vi "Dresden Edit Recipe(in).vi"() -> ()   [LabVIEW 2009] (continued)
              n372 = local write "R_Recipe_type_selection"(enum32{"Single Recipe", "Combination Sputter"}."Combination Sputter" ("R_Recipe_type_selection")) -> ()
              n373 = property on="R Web speed(cm/min)" class="DigNum (strict)"("DisabledEnum"=T5."Disabled and Grayed Out" ("Disabled")) -> ()  [unwired: 2 in, 2 out]
            }
          }
          n374 = Mantissa & Exponent(0:w608) -> (2:w601:dbl)  [unwired: 1 out]
          n375 = Equal?(x="Active", y=w267) -> (x = y?=w269:bool)
          n376 = local write "R_Target Thickness Value"(w495) -> ()
          n377 = local write "R_Duration"(w494) -> ()
          n378 = local write "R Maximum diameter"(w500) -> ()
          n379 = local write "R Minimum diameter"(w501) -> ()
          n380 = local write "R Web thickness"(w499) -> ()
          n381 = local write "R Web speed(cm/min)"(w498) -> ()
          n382 = local write "R Tension Value"(w497) -> ()
          n383 = local write "R  Total length"(w496) -> ()
          n384 = case shown="True" w269 {
            frame #0 {
              n385 = local write "R Single DC Step2 Coating Power Active"(FALSE ("R Single DC Step1 Coating Power Active")) -> ()
            }
            frame #1 {
              n386 = local write "R Single DC Step2 Coating Power Active"(TRUE ("R Single DC Step1 Coating Power Active")) -> ()
            }
          }
          n387 = case shown="True" w271 {
            frame #0 {
              n388 = local write "R Single DC Step1 Coating Power Active"(FALSE ("R Single DC Step1 Coating Power Active")) -> ()
            }
            frame #1 {
              n389 = local write "R Single DC Step1 Coating Power Active"(TRUE ("R Single DC Step1 Coating Power Active")) -> ()
            }
          }
          n390 = case shown="1" w601 {
            frame #0 {
            }
            frame #1 {
              n391 = local write "R_DC_Chamber_selection"(enum32{"Chamber II", "Chamber III"}."Chamber II" ("R_DC_Chamber_selection")) -> ()
            }
            frame #2 {
              n392 = local write "R_DC_Chamber_selection"(enum32{"Chamber II", "Chamber III"}."Chamber III" ("R_DC_Chamber_selection")) -> ()
            }
          }
          n393 = stacked-sequence {
            frame #0 {
            }
          }
          n394 = stacked-sequence {
            frame #0 {
            }
          }
          n395 = stacked-sequence {
            frame #0 {
            }
          }
          n396 = stacked-sequence {
            frame #0 {
              # "Recipe Parameters"
            }
          }
        }
        frame #1 {
        }
      }
    }
    frame #4 {
      n397 = local read "Recipe_cancel"() -> (w818:bool)
      n398 = case shown="False" w818 {
        frame #0 {
          n399 = Wait (ms)(milliseconds to wait=u32 1000) -> ()  [unwired: 1 out]
        }
        frame #1 {
        }
      }
    }
    frame #5 {
      n400 = local read "Recipe_cancel"() -> (w821:bool)
      n401 = case shown="False" w821 {
        tunnel: [w822 FALSE] -> w820
        frame #0 {
          n402 = while {
            tunnel: [w851] -> w822
            stop <- w851 stop-if-true
            n403 = local read "R Single DC Step1 Coating Power Active"() -> (w850:bool)
            n404 = local read "R Single RF Step4 Coating Power Active"() -> (w838:bool)
            n405 = local read "R Single DC Step4 Coating Power Active"() -> (w847:bool)
            n406 = local read "R Single DC Step2 Coating Power Active"() -> (w849:bool)
            n407 = local read "R Single RF Step3 Coating Power Active"() -> (w839:bool)
            n408 = local read "R Single RF Step1 Coating Power Active"() -> (w841:bool)
            n409 = local read "R Single DC Step3 Coating Power Active"() -> (w848:bool)
            n410 = local read "R Single RF Step5 Coating Power Active"() -> (w837:bool)
            n411 = local read "R Single RF Step9 Coating Power Active"() -> (w836:bool)
            n412 = local read "R_Recipe_type_selection"() -> (w823:enum32{"Single Recipe", "Combination Sputter"})
            n413 = local read "R Single RF Step2 Coating Power Active"() -> (w840:bool)
            n414 = case shown="\"Combination Sputter\"" w823 {
              frame #0 {
                n415 = local read "Web_selection_tab"() -> (w1019:T4)
                n416 = Equal?(x=w1019, y=0) -> (x = y?=w1018:bool)
                n417 = case shown="True" w1018 {
                  frame #0 {
                  }
                  frame #1 {
                    w1021 = T5."Enabled" ("Disabled")
                    n418 = property on="R Minimum diameter" class="DigNum (strict)"("DisabledEnum"=w1021) -> ()  [unwired: 2 in, 2 out]
                    n419 = property on="R Maximum diameter" class="DigNum (strict)"("DisabledEnum"=w1021) -> ()  [unwired: 2 in, 2 out]
                    n420 = property on="R Web thickness" class="DigNum (strict)"("DisabledEnum"=w1021) -> ()  [unwired: 2 in, 2 out]
                    n421 = property on="R Web speed(cm/min)" class="DigNum (strict)"("DisabledEnum"=w1021) -> ()  [unwired: 2 in, 2 out]
                    n422 = property on="R Tension Value" class="DigNum (strict)"("DisabledEnum"=w1021) -> ()  [unwired: 2 in, 2 out]
                    n423 = property on="R_Single Microwave Time" class="DigNum (strict)"("DisabledEnum"=T5."Disabled and Grayed Out" ("Disabled")) -> ()  [unwired: 2 in, 2 out]
                  }
                }
              }
              frame #1 {
                n424 = local read "R_Web_selection"() -> (w1024:enum32{"Web", "Other"})
                n425 = Equal?(x=w1024, y=0) -> (x = y?=w1025:bool)
                n426 = case shown="True" w1025 {
                  frame #0 {
                  }
                  frame #1 {
                    w1027 = T5."Enabled" ("Disabled")
                    n427 = local write "R Web speed(cm/min)"(0.0 ("R Web speed(cm/min)")) -> ()
                    n428 = property on="R Tension Value" class="DigNum (strict)"("DisabledEnum"=w1027) -> ()  [unwired: 2 in, 2 out]
                    n429 = property on="R Minimum diameter" class="DigNum (strict)"("DisabledEnum"=w1027) -> ()  [unwired: 2 in, 2 out]
                    n430 = property on="R Maximum diameter" class="DigNum (strict)"("DisabledEnum"=w1027) -> ()  [unwired: 2 in, 2 out]
                    n431 = property on="R Web thickness" class="DigNum (strict)"("DisabledEnum"=w1027) -> ()  [unwired: 2 in, 2 out]
                    n432 = property on="R Web speed(cm/min)" class="DigNum (strict)"("DisabledEnum"=T5."Disabled and Grayed Out" ("Disabled")) -> ()  [unwired: 2 in, 2 out]
                  }
                }
              }
            }
            n433 = case shown="True" w850 {
              frame #0 {
              }
              frame #1 {
                n434 = local read "R Single DC Step2 Coating Power Active"() -> (w1157:bool)
                n435 = case shown="False" w1157 {
                  frame #0 {
                    w1158 = 0.0 ("Target Clean Power")
                    w1159 = T5."Disabled and Grayed Out" ("Disabled")
                    n436 = local write "R Single DC Step2 Coating Power"(w1158) -> ()
                    n437 = local write "R Single DC Interval length2"(w1158) -> ()
                    n438 = property on="R Single DC Interval length2" class="DigNum (strict)"("DisabledEnum"=w1159) -> ()  [unwired: 2 in, 2 out]
                    n439 = property on="R Single DC Step2 Coating Power" class="DigNum (strict)"("DisabledEnum"=w1159) -> ()  [unwired: 2 in, 2 out]
                  }
                  frame #1 {
                    w1160 = T5."Enabled" ("Disabled")
                    n440 = property on="R Single DC Step2 Coating Power" class="DigNum (strict)"("DisabledEnum"=w1160) -> ()  [unwired: 2 in, 2 out]
                    n441 = property on="R Single DC Interval length2" class="DigNum (strict)"("DisabledEnum"=w1160) -> ()  [unwired: 2 in, 2 out]
                  }
                }
              }
            }
            n442 = local read "R_Recipe_type_selection"() -> (w989:enum32{"Single Recipe", "Combination Sputter"})
            n443 = case shown="False" w838 {
              frame #0 {
                w1098 = FALSE ("R Single RF Step3 Coating Power Active")
                n444 = local write "R Single RF Step5 Coating Power Active"(w1098) -> ()
                n445 = local write "R Single RF Step6 Coating Power Active"(w1098) -> ()
                n446 = local write "R Single RF Step7 Coating Power Active"(w1098) -> ()
                n447 = local write "R Single RF Step8 Coating Power Active"(w1098) -> ()
                n448 = local write "R Single RF Step9 Coating Power Active"(w1098) -> ()
                n449 = local write "R Single RF Step10 Coating Power Active"(w1098) -> ()
              }
              frame #1 {
                n450 = local read "R Single RF Step5 Coating Power Active"() -> (w1099:bool)
                n451 = case shown="False" w1099 {
                  frame #0 {
                    w1101 = T5."Disabled and Grayed Out" ("Disabled")
                    w1100 = 0.0 ("Target Clean Power")
                    n452 = local write "R Single RF Step5 Coating Power"(w1100) -> ()
                    n453 = local write "R Single RF Interval length5"(w1100) -> ()
                    n454 = property on="R Single RF Interval length5" class="DigNum (strict)"("DisabledEnum"=w1101) -> ()  [unwired: 2 in, 2 out]
                    n455 = property on="R Single RF Step5 Coating Power" class="DigNum (strict)"("DisabledEnum"=w1101) -> ()  [unwired: 2 in, 2 out]
                  }
                  frame #1 {
                    w1102 = T5."Enabled" ("Disabled")
                    n456 = property on="R Single RF Step5 Coating Power" class="DigNum (strict)"("DisabledEnum"=w1102) -> ()  [unwired: 2 in, 2 out]
                    n457 = property on="R Single RF Interval length5" class="DigNum (strict)"("DisabledEnum"=w1102) -> ()  [unwired: 2 in, 2 out]
                  }
                }
              }
            }
            n458 = local read "R_Recipe_type_selection"() -> (w858:enum32{"Single Recipe", "Combination Sputter"})
            n459 = case shown="False" w839 {
              frame #0 {
                w1103 = FALSE ("R Single RF Step3 Coating Power Active")
                n460 = local write "R Single RF Step4 Coating Power Active"(w1103) -> ()
                n461 = local write "R Single RF Step5 Coating Power Active"(w1103) -> ()
                n462 = local write "R Single RF Step6 Coating Power Active"(w1103) -> ()
                n463 = local write "R Single RF Step7 Coating Power Active"(w1103) -> ()
                n464 = local write "R Single RF Step8 Coating Power Active"(w1103) -> ()
                n465 = local write "R Single RF Step9 Coating Power Active"(w1103) -> ()
                n466 = local write "R Single RF Step10 Coating Power Active"(w1103) -> ()
              }
              frame #1 {
                n467 = local read "R Single RF Step4 Coating Power Active"() -> (w1104:bool)
                n468 = case shown="False" w1104 {
                  frame #0 {
                    w1106 = T5."Disabled and Grayed Out" ("Disabled")
                    w1105 = 0.0 ("Target Clean Power")
                    n469 = local write "R Single RF Interval length4"(w1105) -> ()
                    n470 = local write "R Single RF Step4 Coating Power"(w1105) -> ()
                    n471 = property on="R Single RF Step4 Coating Power" class="DigNum (strict)"("DisabledEnum"=w1106) -> ()  [unwired: 2 in, 2 out]
                    n472 = property on="R Single RF Interval length4" class="DigNum (strict)"("DisabledEnum"=w1106) -> ()  [unwired: 2 in, 2 out]
                  }
                  frame #1 {
                    w1107 = T5."Enabled" ("Disabled")
                    n473 = property on="R Single RF Step4 Coating Power" class="DigNum (strict)"("DisabledEnum"=w1107) -> ()  [unwired: 2 in, 2 out]
                    n474 = property on="R Single RF Interval length4" class="DigNum (strict)"("DisabledEnum"=w1107) -> ()  [unwired: 2 in, 2 out]
                  }
                }
              }
            }
            n475 = case shown="False" w849 {
              frame #0 {
                w1152 = FALSE ("R Single DC Step8 Coating Power Active")
                n476 = local write "R Single DC Step7 Coating Power Active"(w1152) -> ()
                n477 = local write "R Single DC Step8 Coating Power Active"(w1152) -> ()
                n478 = local write "R Single DC Step9 Coating Power Active"(w1152) -> ()
                n479 = local write "R Single DC Step10 Coating Power Active"(w1152) -> ()
                n480 = local write "R Single DC Step6 Coating Power Active"(w1152) -> ()
                n481 = local write "R Single DC Step3 Coating Power Active"(w1152) -> ()
                n482 = local write "R Single DC Step4 Coating Power Active"(w1152) -> ()
                n483 = local write "R Single DC Step5 Coating Power Active"(w1152) -> ()
              }
              frame #1 {
                n484 = local read "R Single DC Step3 Coating Power Active"() -> (w1153:bool)
                n485 = case shown="False" w1153 {
                  frame #0 {
                    w1154 = 0.0 ("Target Clean Power")
                    w1155 = T5."Disabled and Grayed Out" ("Disabled")
                    n486 = local write "R Single DC Step3 Coating Power"(w1154) -> ()
                    n487 = local write "R Single DC Interval length3"(w1154) -> ()
                    n488 = property on="R Single DC Interval length3" class="DigNum (strict)"("DisabledEnum"=w1155) -> ()  [unwired: 2 in, 2 out]
                    n489 = property on="R Single DC Step3 Coating Power" class="DigNum (strict)"("DisabledEnum"=w1155) -> ()  [unwired: 2 in, 2 out]
                  }
                  frame #1 {
                    w1156 = T5."Enabled" ("Disabled")
                    n490 = property on="R Single DC Step3 Coating Power" class="DigNum (strict)"("DisabledEnum"=w1156) -> ()  [unwired: 2 in, 2 out]
                    n491 = property on="R Single DC Interval length3" class="DigNum (strict)"("DisabledEnum"=w1156) -> ()  [unwired: 2 in, 2 out]
                  }
                }
              }
            }
            n492 = case shown="False" w847 {
              frame #0 {
                w1142 = FALSE ("R Single DC Step8 Coating Power Active")
                n493 = local write "R Single DC Step7 Coating Power Active"(w1142) -> ()
                n494 = local write "R Single DC Step8 Coating Power Active"(w1142) -> ()
                n495 = local write "R Single DC Step9 Coating Power Active"(w1142) -> ()
                n496 = local write "R Single DC Step10 Coating Power Active"(w1142) -> ()
                n497 = local write "R Single DC Step5 Coating Power Active"(w1142) -> ()
                n498 = local write "R Single DC Step6 Coating Power Active"(w1142) -> ()
              }
              frame #1 {
                n499 = local read "R Single DC Step5 Coating Power Active"() -> (w1143:bool)
                n500 = case shown="False" w1143 {
                  frame #0 {
                    w1144 = 0.0 ("Target Clean Power")
                    w1145 = T5."Disabled and Grayed Out" ("Disabled")
                    n501 = local write "R Single DC Step5 Coating Power"(w1144) -> ()
                    n502 = local write "R Single DC Interval length5"(w1144) -> ()
                    n503 = property on="R Single DC Step5 Coating Power" class="DigNum (strict)"("DisabledEnum"=w1145) -> ()  [unwired: 2 in, 2 out]
                    n504 = property on="R Single DC Interval length5" class="DigNum (strict)"("DisabledEnum"=w1145) -> ()  [unwired: 2 in, 2 out]
                  }
                  frame #1 {
                    w1146 = T5."Enabled" ("Disabled")
                    n505 = property on="R Single DC Step5 Coating Power" class="DigNum (strict)"("DisabledEnum"=w1146) -> ()  [unwired: 2 in, 2 out]
                    n506 = property on="R Single DC Interval length5" class="DigNum (strict)"("DisabledEnum"=w1146) -> ()  [unwired: 2 in, 2 out]
                  }
                }
              }
            }
            n507 = case shown="False" w848 {
              frame #0 {
                w1147 = FALSE ("R Single DC Step8 Coating Power Active")
                n508 = local write "R Single DC Step7 Coating Power Active"(w1147) -> ()
                n509 = local write "R Single DC Step8 Coating Power Active"(w1147) -> ()
                n510 = local write "R Single DC Step9 Coating Power Active"(w1147) -> ()
                n511 = local write "R Single DC Step10 Coating Power Active"(w1147) -> ()
                n512 = local write "R Single DC Step6 Coating Power Active"(w1147) -> ()
                n513 = local write "R Single DC Step5 Coating Power Active"(w1147) -> ()
                n514 = local write "R Single DC Step4 Coating Power Active"(w1147) -> ()
              }
              frame #1 {
                n515 = local read "R Single DC Step4 Coating Power Active"() -> (w1148:bool)
                n516 = case shown="False" w1148 {
                  frame #0 {
                    w1149 = 0.0 ("Target Clean Power")
                    w1150 = T5."Disabled and Grayed Out" ("Disabled")
                    n517 = local write "R Single DC Step4 Coating Power"(w1149) -> ()
                    n518 = local write "R Single DC Interval length4"(w1149) -> ()
                    n519 = property on="R Single DC Step4 Coating Power" class="DigNum (strict)"("DisabledEnum"=w1150) -> ()  [unwired: 2 in, 2 out]
                    n520 = property on="R Single DC Interval length4" class="DigNum (strict)"("DisabledEnum"=w1150) -> ()  [unwired: 2 in, 2 out]
                  }
                  frame #1 {
                    w1151 = T5."Enabled" ("Disabled")
                    n521 = property on="R Single DC Step4 Coating Power" class="DigNum (strict)"("DisabledEnum"=w1151) -> ()  [unwired: 2 in, 2 out]
                    n522 = property on="R Single DC Interval length4" class="DigNum (strict)"("DisabledEnum"=w1151) -> ()  [unwired: 2 in, 2 out]
                  }
                }
              }
            }
            n523 = case shown="True" w841 {
              frame #0 {
              }
              frame #1 {
                n524 = local read "R Single RF Step2 Coating Power Active"() -> (w1113:bool)
                n525 = case shown="False" w1113 {
                  frame #0 {
                    w1115 = T5."Disabled and Grayed Out" ("Disabled")
                    w1114 = 0.0 ("Target Clean Power")
                    n526 = local write "R Single RF Step2 Coating Power"(w1114) -> ()
                    n527 = local write "R Single RF Interval length2"(w1114) -> ()
                    n528 = property on="R Single RF Step2 Coating Power" class="DigNum (strict)"("DisabledEnum"=w1115) -> ()  [unwired: 2 in, 2 out]
                    n529 = property on="R Single RF Interval length2" class="DigNum (strict)"("DisabledEnum"=w1115) -> ()  [unwired: 2 in, 2 out]
                  }
                  frame #1 {
                    w1116 = T5."Enabled" ("Disabled")
                    n530 = property on="R Single RF Step2 Coating Power" class="DigNum (strict)"("DisabledEnum"=w1116) -> ()  [unwired: 2 in, 2 out]
                    n531 = property on="R Single RF Interval length2" class="DigNum (strict)"("DisabledEnum"=w1116) -> ()  [unwired: 2 in, 2 out]
                  }
                }
              }
            }
            n532 = local read "R Single RF Step1 Coating Power Active"() -> (w997:bool)
            n533 = case shown="False" w840 {
              frame #0 {
                w1108 = FALSE ("R Single RF Step3 Coating Power Active")
                n534 = local write "R Single RF Step3 Coating Power Active"(w1108) -> ()
                n535 = local write "R Single RF Step4 Coating Power Active"(w1108) -> ()
                n536 = local write "R Single RF Step5 Coating Power Active"(w1108) -> ()
                n537 = local write "R Single RF Step6 Coating Power Active"(w1108) -> ()
                n538 = local write "R Single RF Step7 Coating Power Active"(w1108) -> ()
                n539 = local write "R Single RF Step8 Coating Power Active"(w1108) -> ()
                n540 = local write "R Single RF Step9 Coating Power Active"(w1108) -> ()
                n541 = local write "R Single RF Step10 Coating Power Active"(w1108) -> ()
              }
              frame #1 {
                n542 = local read "R Single RF Step3 Coating Power Active"() -> (w1109:bool)
                n543 = case shown="False" w1109 {
                  frame #0 {
                    w1111 = T5."Disabled and Grayed Out" ("Disabled")
                    w1110 = 0.0 ("Target Clean Power")
                    n544 = local write "R Single RF Step3 Coating Power"(w1110) -> ()
                    n545 = local write "R Single RF Interval length3"(w1110) -> ()
                    n546 = property on="R Single RF Step3 Coating Power" class="DigNum (strict)"("DisabledEnum"=w1111) -> ()  [unwired: 2 in, 2 out]
                    n547 = property on="R Single RF Interval length3" class="DigNum (strict)"("DisabledEnum"=w1111) -> ()  [unwired: 2 in, 2 out]
                  }
                  frame #1 {
                    w1112 = T5."Enabled" ("Disabled")
                    n548 = property on="R Single RF Step3 Coating Power" class="DigNum (strict)"("DisabledEnum"=w1112) -> ()  [unwired: 2 in, 2 out]
                    n549 = property on="R Single RF Interval length3" class="DigNum (strict)"("DisabledEnum"=w1112) -> ()  [unwired: 2 in, 2 out]
                  }
                }
              }
            }
            n550 = case shown="False" w837 {
              frame #0 {
                w1093 = FALSE ("R Single RF Step3 Coating Power Active")
                n551 = local write "R Single RF Step6 Coating Power Active"(w1093) -> ()
                n552 = local write "R Single RF Step7 Coating Power Active"(w1093) -> ()
                n553 = local write "R Single RF Step8 Coating Power Active"(w1093) -> ()
                n554 = local write "R Single RF Step9 Coating Power Active"(w1093) -> ()
                n555 = local write "R Single RF Step10 Coating Power Active"(w1093) -> ()
              }
              frame #1 {
                n556 = local read "R Single RF Step6 Coating Power Active"() -> (w1094:bool)
                n557 = case shown="False" w1094 {
                  frame #0 {
                    w1095 = 0.0 ("Target Clean Power")
                    w1096 = T5."Disabled and Grayed Out" ("Disabled")
                    n558 = property on="R Single RF Interval length6" class="DigNum (strict)"("DisabledEnum"=w1096) -> ()  [unwired: 2 in, 2 out]
                    n559 = property on="R Single RF Step6 Coating Power" class="DigNum (strict)"("DisabledEnum"=w1096) -> ()  [unwired: 2 in, 2 out]
                    n560 = local write "R Single RF Step6 Coating Power"(w1095) -> ()
                    n561 = local write "R Single RF Interval length6"(w1095) -> ()
                  }
                  frame #1 {
                    w1097 = T5."Enabled" ("Disabled")
                    n562 = property on="R Single RF Step6 Coating Power" class="DigNum (strict)"("DisabledEnum"=w1097) -> ()  [unwired: 2 in, 2 out]
                    n563 = property on="R Single RF Interval length6" class="DigNum (strict)"("DisabledEnum"=w1097) -> ()  [unwired: 2 in, 2 out]
                  }
                }
              }
            }
            n564 = case shown="False" w836 {
              frame #0 {
                n565 = local write "R Single RF Step10 Coating Power Active"(FALSE ("R Single RF Step3 Coating Power Active")) -> ()
              }
              frame #1 {
                n566 = local read "R Single RF Step10 Coating Power Active"() -> (w1089:bool)
                n567 = case shown="False" w1089 {
                  frame #0 {
                    w1090 = 0.0 ("Target Clean Power")
                    w1091 = T5."Disabled and Grayed Out" ("Disabled")
                    n568 = local write "R Single RF Step10 Coating Power"(w1090) -> ()
                    n569 = local write "R Single RF Interval length10"(w1090) -> ()
                    n570 = property on="R Single RF Step10 Coating Power" class="DigNum (strict)"("DisabledEnum"=w1091) -> ()  [unwired: 2 in, 2 out]
                    n571 = property on="R Single RF Interval length10" class="DigNum (strict)"("DisabledEnum"=w1091) -> ()  [unwired: 2 in, 2 out]
                  }
                  frame #1 {
                    w1092 = T5."Enabled" ("Disabled")
                    n572 = property on="R Single RF Step10 Coating Power" class="DigNum (strict)"("DisabledEnum"=w1092) -> ()  [unwired: 2 in, 2 out]
                    n573 = property on="R Single RF Interval length10" class="DigNum (strict)"("DisabledEnum"=w1092) -> ()  [unwired: 2 in, 2 out]
                  }
                }
              }
            }
            n574 = local read "R_Simple_Coating Type Selection"() -> (w1005:T2)
            n575 = local read "R Single DC Step1 Coating Power Active"() -> (w998:bool)
            n576 = local read "R_Web_selection"() -> (w1010:enum32{"Web", "Other"})
            n577 = local read "R_Recipe_type_selection"() -> (w1006:enum32{"Single Recipe", "Combination Sputter"})
            n578 = Wait Until Next ms Multiple(millisecond multiple=u32 50) -> ()  [unwired: 1 out]
            n579 = local read "R Single DC Step1 Coating Power Active"() -> (w981:bool)
            n580 = local read "R Single DC Step4 Coating Power Active"() -> (w973:bool)
            n581 = local read "R Single DC Step3 Coating Power Active"() -> (w975:bool)
            n582 = local read "R Single DC Step2 Coating Power Active"() -> (w979:bool)
            n583 = local read "R Single DC Step5 Coating Power Active"() -> (w965:bool)
            n584 = local read "R Single DC Step6 Coating Power Active"() -> (w964:bool)
            n585 = local read "R Single DC Step7 Coating Power Active"() -> (w963:bool)
            n586 = local read "R Single DC Step10 Coating Power Active"() -> (w960:bool)
            n587 = local read "R Single RF Step7 Coating Power Active"() -> (w925:bool)
            n588 = local read "R Single DC Step8 Coating Power Active"() -> (w962:bool)
            n589 = local read "R Single DC Step9 Coating Power Active"() -> (w961:bool)
            n590 = local read "R Single RF Step9 Coating Power Active"() -> (w923:bool)
            n591 = local read "R Single RF Step10 Coating Power Active"() -> (w922:bool)
            n592 = local read "R Single RF Ramp up"() -> (w995:bool)
            n593 = local read "R Single RF Step1 Coating Power Active"() -> (w940:bool)
            n594 = local read "R Single RF Step2 Coating Power Active"() -> (w930:bool)
            n595 = local read "R Single RF Step3 Coating Power Active"() -> (w929:bool)
            n596 = local read "R Single RF Step4 Coating Power Active"() -> (w928:bool)
            n597 = local read "R Single RF Step5 Coating Power Active"() -> (w927:bool)
            n598 = local read "R Single RF Step6 Coating Power Active"() -> (w926:bool)
            n599 = local read "R Single RF Step8 Coating Power Active"() -> (w924:bool)
            n600 = local read "R Single RF Ramp down"() -> (w996:bool)
            n601 = Equal?(x=w989, y=0) -> (x = y?=w859:bool)
            n602 = Equal?(x=w858, y=1) -> (x = y?=w856:bool)
            n603 = case shown="True" "OK" {
              tunnel: [FALSE w1310] -> w853
              frame #0 {
              }
              frame #1 {
                # "TENSION IS NOT LOWER THAN 5\nTENSION IS NOT BIGGER THAN10"
                # "92"
                # "91"
                # "2"
                # "1"
                n604 = local read "R_Web_selection"() -> (w1306:enum32{"Web", "Other"})
                n605 = local read "R_Recipe_type_selection"() -> (w1328:enum32{"Single Recipe", "Combination Sputter"})
                n606 = local read "R_Recipe_type_selection"() -> (w1343:enum32{"Single Recipe", "Combination Sputter"})
                n607 = local read "R_Recipe_type_selection"() -> (w1340:enum32{"Single Recipe", "Combination Sputter"})
                n608 = local read "Substrate Material"() -> (w1348:string)
                n609 = local read "Recipe Name"() -> (w1347:string)
                n610 = Equal?(x=w1306, y=1) -> (x = y?=w1304:bool)
                n611 = Equal?(x=w1348, y="") -> (x = y?=w1314:bool)
                n612 = Equal?(x=w1328, y=0) -> (x = y?=w1330:bool)
                n613 = Equal?(x=w1347, y="") -> (x = y?=w1349:bool)
                n614 = Equal?(x=w1343, y=0) -> (x = y?=w1342:bool)
                n615 = Equal?(x=w1340, y=0) -> (x = y?=w1338:bool)
                n616 = case shown="True" w1304 {
                  tunnel: [FALSE w1539] -> w1303
                  frame #0 {
                  }
                  frame #1 {
                    n617 = local read "R_Simple_Coating Type Selection"() -> (w1540:T2)
                    n618 = Equal?(x=w1540, y=0) -> (x = y?=w1539:bool)
                  }
                }
                n619 = case shown="True" w1330 {
                  tunnel: [FALSE w1640] -> w1331
                  frame #0 {
                  }
                  frame #1 {
                    n620 = local read "R_Simple_Coating Type Selection"() -> (w1641:T2)
                    n621 = Equal?(x=w1641, y=2) -> (x = y?=w1640:bool)
                  }
                }
                n622 = case shown="True" w1342 {
                  tunnel: [FALSE w1691] -> w1341
                  frame #0 {
                  }
                  frame #1 {
                    n623 = local read "R_Simple_Coating Type Selection"() -> (w1692:T2)
                    n624 = Equal?(x=w1692, y=0) -> (x = y?=w1691:bool)
                  }
                }
                n625 = case shown="True" w1338 {
                  tunnel: [FALSE w1681] -> w1337
                  frame #0 {
                  }
                  frame #1 {
                    n626 = local read "R_Simple_Coating Type Selection"() -> (w1682:T2)
                    n627 = Equal?(x=w1682, y=1) -> (x = y?=w1681:bool)
                  }
                }
                n628 = local read "R Single RF Step1 Coating Power Active"() -> (w1326:bool)
                n629 = local read "R Single RF Step4 Coating Power Active"() -> (w1308:bool)
                n630 = local read "R Single RF Step2 Coating Power Active"() -> (w1325:bool)
                n631 = local read "R Single DC Step6 Coating Power Active"() -> (w1302:bool)
                n632 = local read "R Single DC Step5 Coating Power Active"() -> (w1332:bool)
                n633 = local read "R Single DC Step8 Coating Power Active"() -> (w1300:bool)
                n634 = local read "R Single RF Step3 Coating Power Active"() -> (w1309:bool)
                n635 = local read "R Single DC Step2 Coating Power Active"() -> (w1335:bool)
                n636 = local read "R Single DC Step4 Coating Power Active"() -> (w1333:bool)
                n637 = local read "R Single DC Step1 Coating Power Active"() -> (w1336:bool)
                n638 = local read "R Single DC Step7 Coating Power Active"() -> (w1301:bool)
                n639 = local read "R Single DC Step10 Coating Power Active"() -> (w1179:bool)
                n640 = local read "R Single RF Step6 Coating Power Active"() -> (w1298:bool)
                n641 = local read "R Single RF Step7 Coating Power Active"() -> (w1297:bool)
                n642 = local read "R Single DC Step3 Coating Power Active"() -> (w1334:bool)
                n643 = local read "R Single RF Step5 Coating Power Active"() -> (w1324:bool)
                n644 = local read "R Single DC Step9 Coating Power Active"() -> (w1299:bool)
                n645 = local read "R Single RF Step8 Coating Power Active"() -> (w1296:bool)
                n646 = local read "R Single RF Ramp up"() -> (w1327:bool)
                n647 = case shown="True" w1332 {
                  tunnel: [FALSE w1648] -> w1269
                  tunnel: [FALSE w1645] -> w1268
                  frame #0 {
                  }
                  frame #1 {
                    # "17"
                    # "16"
                    n648 = local read "R Single DC Step5 Coating Power"() -> (w1647:dbl)
                    n649 = local read "R Single DC Interval length5"() -> (w1646:dbl)
                    n650 = Equal To 0?(x=w1647) -> (x = 0?=w1648:bool)
                    n651 = Equal To 0?(x=w1646) -> (x = 0?=w1645:bool)
                  }
                }
                n652 = case shown="True" w1299 {
                  tunnel: [FALSE w1516] -> w1261
                  tunnel: [FALSE w1515] -> w1260
                  frame #0 {
                  }
                  frame #1 {
                    # "25"
                    # "24"
